vi "Launch Plugin.vi"(8 "error in (no error)":errorcluster, 9 "Open Actor Core front panel? (F)":bool, 10 "Plugin.lvclass":refnum<class "Plugin.lvclass">, 11 "Management in":refnum<class "Display.lvclass">) -> (0 "error out":errorcluster, 3 "Management out":refnum<class "Display.lvclass">)   [LabVIEW 2015, in "UserManagement.lvlib" / "Display.lvclass"]
uses:
  Display.lvclass
  Plugin/Plugin.lvclass
  Display.lvclass/Display.ctl
  Plugin/Plugin.lvclass/Plugin.ctl
  <vilib>/ActorFramework/Actor/Actor.lvclass
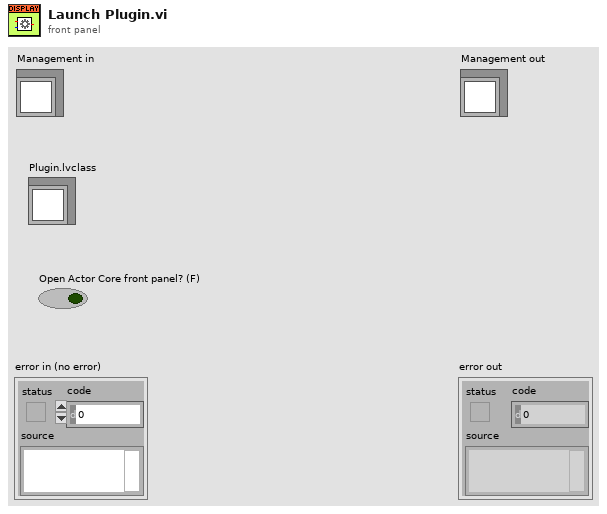
[diagram p1: front panel]
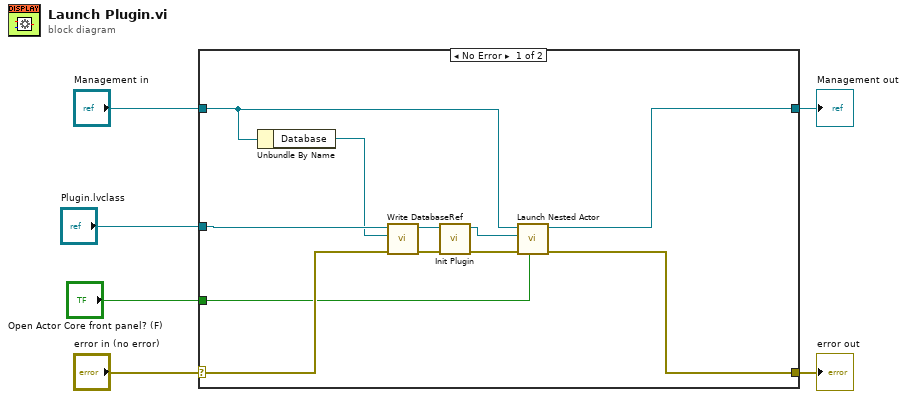
[diagram p0: block diagram]
diagram:
  n1 = case shown="No Error" "error in (no error)" {
    selector: "error in (no error)" -> [w15 w19]
    tunnel: [w13 w19] -> w5
    tunnel: [w12 w18] -> w3
    tunnel: "Management in" -> [w14 w18]
    tunnel: "Plugin.lvclass" -> [w17 _]
    tunnel: "Open Actor Core front panel? (F)" -> [w11 _]
    frame No Error {
      n2 = Unbundle By Name(w14) -> ("Database"=w16:refnum<class "Database.lvclass">)
      n3 = call "Write DatabaseRef.vi"("error in (no error)"=w15, "Database.lvlib:Database"=w16, "Plugin in"=w17) -> ("error out"=w10:errorcluster, "Plugin out"=w9:refnum<class "Plugin.lvclass">)  [unwired: 7 in]
      n4 = call-dynamic "Init Plugin.vi"("error in (no error)"=w10, "Plugin in"=w9) -> ("error out"=w7:errorcluster, "Plugin out"=w8:refnum<class "Plugin.lvclass">)  [unwired: 8 in]
      n5 = call <vilib>:"Launch Nested Actor.vi"("Open Actor Core front panel? (F)"=w11, "error in (no error)"=w7, "Nested Actor"=w8, "Caller Actor in"=w14) -> ("error out"=w13:errorcluster, "Caller Actor out"=w12:refnum<class "Display.lvclass">)  [unwired: 5 in, 1 out]
    }
    frame Error {
    }
  }
  "error out" <- w5
  "Management out" <- w3
